vi "Scale Byte Exp.vi"(9 "Brightness":u8, 10 "Factor":dbl, 11 "Byte":u8) -> (3 "Byte Scaled":u8)   [LabVIEW 2013]
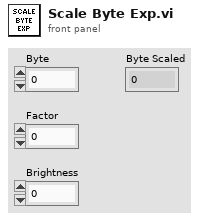
[diagram p1: front panel]
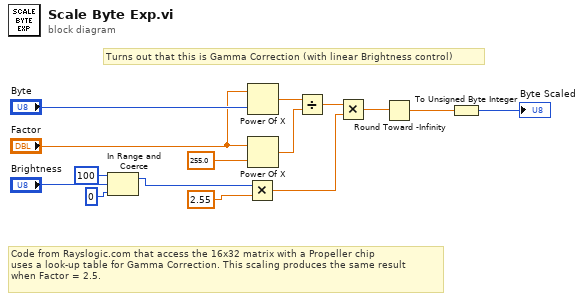
[diagram p0: block diagram]
diagram:
  # "Code from Rayslogic.com that access the 16x32 matrix with a Propeller chip\nuses a look-up table for Gamma Correction. This scaling produces the same result\nwhen Factor = 2.5."
  # "Turns out that this is Gamma Correction (with linear Brightness control)"
  n1 = In Range and Coerce(upper limit=u8 100, x="Brightness", lower limit=u8 0) -> (coerced(x)=w8:u8)  [unwired: 1 out]
  n2 = Multiply(x=w8, y=2.55) -> (x*y=w13:dbl)
  n3 = Power Of X(1:"Byte", 2:"Factor") -> (0:w14:dbl)
  n4 = Power Of X(1:255.0 ("y"), 2:"Factor") -> (0:w15:dbl)
  n5 = Divide(x=w14, y=w15) -> (x/y=w3:dbl)
  n6 = Multiply(x=w3, y=w13) -> (x*y=w2:dbl)
  n7 = Round Toward -Infinity(1:w2) -> (0:w1:dbl)
  n8 = To Unsigned Byte Integer(number=w1) -> (unsigned 8bit integer=→"Byte Scaled":u8)
